vi "Next.vi"(7 "Address":string, 8 "Error In":errorcluster) -> (0 "Error Out":errorcluster)   [LabVIEW 2018, in "Tests.lvlib" / "KnownHosts.lvlib"]
uses:
  KnownHosts.lvlib
  src/Toolkit/API/KnownHosts/API/Typedefs/Get Results.ctl
  <vilib>/Utility/error.llb/Clear Errors.vi
  <vilib>/Utility/file.llb/Is Path and Not Empty.vi
  <vilib>/Utility/sysdir.llb/Get System Directory.vi
  src/Toolkit/API/KnownHost/Support/Create from Known Hosts.vi
  src/Toolkit/API/KnownHost/Support/Destroy to Known Hosts.vi
  <vilib>/addons/_JKI Toolkits/Caraya/classes/Test/Test.lvclass
  <vilib>/addons/_JKI Toolkits/Caraya/classes/Assert/Assert.lvclass
  src/Toolkit/API/KnownHosts/KnownHosts.lvclass
  Tests.lvlib
  src/Toolkit/API/Session/Session.lvclass
  src/Toolkit/API/KnownHost/KnownHost.lvclass
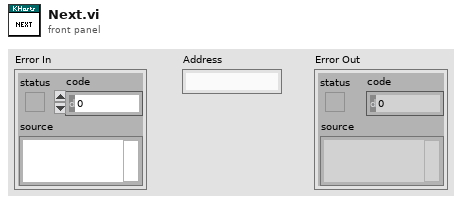
[diagram p1: front panel]
types:
  T1 = typedef "Toolkit.lvlib/KnownHosts.lvclass/Get Results.ctl" = enum32{"Success", "End of Hosts"}
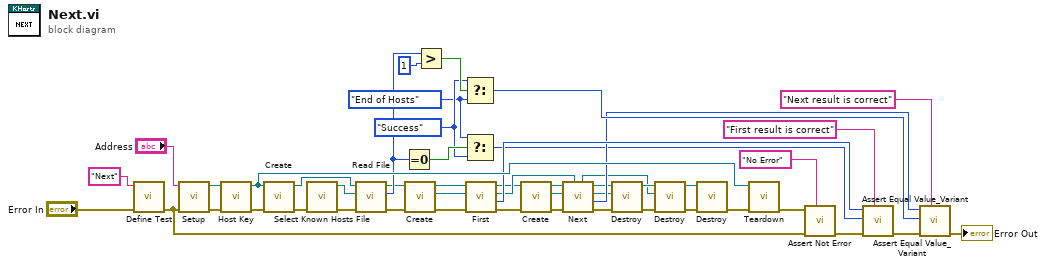
[diagram p0: block diagram]
diagram:
  w15 = Get_Results."End of Hosts" ("Get Result")
  w16 = Get_Results."Success" ("Get Result")
  n1 = call <vilib>:"Define Test.vi"("error in (no error)"="Error In", "Label (VI Title)"="Next") -> ("error out"=w37:errorcluster)  [unwired: 9 in]
  n2 = call "Setup.vi"("Error In"=w37, "Address In"="Address") -> ("Error Out"=w38:errorcluster, "Sesssion"=w39:refnum<class "Session.lvclass">)  [unwired: 7 in, 1 out]
  n3 = call "Host Key.vi"("Error In"=w38, "Session In"=w39) -> ("Error Out"=w40:errorcluster, "Sesssion Out"=w35:refnum<class "Session.lvclass">)  [unwired: 6 in, 2 out]
  n4 = call "Create.vi"("Error In"=w40, "Session"=w35) -> ("Error Out"=w45:errorcluster, "Known Hosts"=w46:refnum<class "KnownHosts.lvclass">)  [unwired: 8 in]
  n5 = call "Select Known Hosts File.vi"("Error In"=w45) -> ("Error Out"=w44:errorcluster, "Known Hosts File"=w43:path)  [unwired: 9 in]
  n6 = call "Read File.vi"("Error In"=w44, "File"=w43, "KnownHosts In"=w46) -> ("Error Out"=w32:errorcluster, "Count"=w19:u64, "KnownHosts Out"=w14:refnum<class "KnownHosts.lvclass">)  [unwired: 6 in]
  n7 = Equal To 0?(x=w19) -> (x = 0?=w18:bool)
  n8 = call-poly "Create.vi"("Error In"=w32, "Known Hosts In"=w14) -> ("Error Out"=w31:errorcluster, "Known Host"=w11:refnum<class "KnownHost.lvclass">, "Known Hosts Out"=w12:refnum<class "KnownHosts.lvclass">)  [unwired: 7 in]
  n9 = Greater?(x=w19, y=u64 1) -> (0:w20:bool)
  n10 = Select(t=w16, s=w20, f=w15) -> (s? t:f=w23:T1)
  n11 = Select(t=w15, s=w18, f=w16) -> (s? t:f=w17:T1)
  n12 = call "First.vi"("Error In"=w31, "Known Host In"=w11, "KnownHosts In"=w12) -> ("Error Out"=w28:errorcluster, "Result"=w30:T1, "Known Host Out"=w29:refnum<class "KnownHost.lvclass">, "KnownHosts Out"=w13:refnum<class "KnownHosts.lvclass">)  [unwired: 5 in]
  n13 = call-poly "Create.vi"("Error In"=w28, "Known Hosts In"=w13) -> ("Error Out"=w27:errorcluster, "Known Host"=w9:refnum<class "KnownHost.lvclass">, "Known Hosts Out"=w10:refnum<class "KnownHosts.lvclass">)  [unwired: 7 in]
  n14 = call "Next.vi"("Previous In"=w29, "Error In"=w27, "Next In"=w9, "KnownHosts In"=w10) -> ("Error Out"=w8:errorcluster, "Result"=w22:T1, "Next Out"=w6:refnum<class "KnownHost.lvclass">, "KnownHosts Out"=w7:refnum<class "KnownHosts.lvclass">, "Previous Out"=w4:refnum<class "KnownHost.lvclass">)  [unwired: 3 in]
  n15 = call-poly "Destroy.vi"("Error In"=w8, "Known Host"=w6, "KnownHosts In"=w7) -> ("Error Out"=w3:errorcluster, "KnownHosts Out"=w5:refnum<class "KnownHosts.lvclass">)  [unwired: 7 in]
  n16 = call-poly "Destroy.vi"("Error In"=w3, "Known Host"=w4, "KnownHosts In"=w5) -> ("Error Out"=w1:errorcluster, "KnownHosts Out"=w2:refnum<class "KnownHosts.lvclass">)  [unwired: 7 in]
  n17 = call "Destroy.vi"("Error In"=w1, "KnownHosts"=w2) -> ("Error Out"=w34:errorcluster)  [unwired: 8 in, 1 out]
  n18 = call "Teardown.vi"("Error In"=w34, "Session"=w35) -> ("Error Out"=w33:errorcluster)  [unwired: 9 in]
  n19 = call <vilib>:"Assert Not Error.vi"("Label"="No Error", "error in (no error)"=w37, "Not Error?"=w33) -> ("error out"=w42:errorcluster)  [unwired: 8 in]
  n20 = call <vilib>:"Assert Equal Value_Variant.vi"("Label"="First result is correct", "error in (no error)"=w42, "Y"=w17, "X"=w30) -> ("error out"=w26:errorcluster)  [unwired: 7 in]
  n21 = call <vilib>:"Assert Equal Value_Variant.vi"("Label"="Next result is correct", "error in (no error)"=w26, "Y"=w23, "X"=w22) -> ("error out"=→"Error Out":errorcluster)  [unwired: 7 in]
